vi "tm_getnextframe_a.vi"(7 "Timeout":i32=-1, 8 "error in (no error)":errorcluster, 10 "Buffer":u16[][](array[numeric]), 11 "Handle in":u32) -> (0 "error out":errorcluster, 2 "Data":u16[][](array[numeric]), 3 "Handle out":u32)   [LabVIEW 2011]
uses:
  tmcamcon.dll
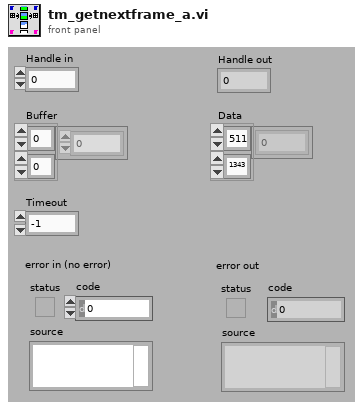
[diagram p1: front panel]
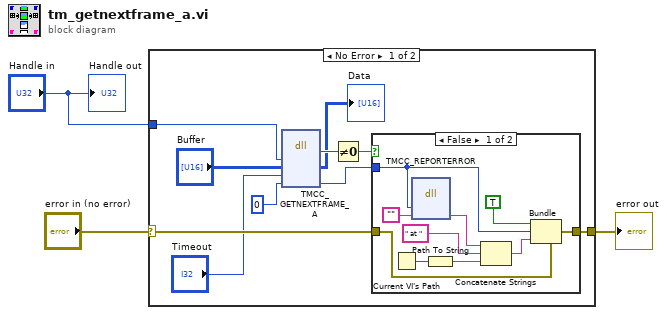
[diagram p0: block diagram]
diagram:
  n1 = case shown="No Error" "error in (no error)" {
    selector: "error in (no error)" -> [w7 w25]
    tunnel: [w6 w25] -> w2
    tunnel: "Handle in" -> [w5 _]
    frame No Error {
      n2 = dll-call lib="tmcamcon.dll" fn="TMCC_GETNEXTFRAME_A"("index"=w5, "imgarray"="Buffer", "timeout"="Timeout", "Erval"=0) -> ("return type"=w13:u32, "imgarray"=→"Data":u16[][], "Erval"=w8:i32)  [unwired: 5 in, 2 out]
      n3 = Not Equal To 0?(x=w13) -> (x != 0?=w9:bool)
      n4 = case shown="False" w9 {
        tunnel: w7 -> [w23 w24]
        tunnel: [w22 w24] -> w6
        tunnel: w8 -> [w16 _]
        frame False {
          n5 = Current VI's Path() -> (path=w21:path)
          n6 = dll-call lib="tmcamcon.dll" fn="TMCC_REPORTERROR"("error"=w16, "buf"="") -> ("buf"=w15:string)  [unwired: 5 in, 2 out]
          n7 = Path To String(path=w21) -> (string=w17:string)
          n8 = Concatenate Strings(w15, " at ", w17) -> (w20:string)
          n9 = Bundle(cluster=w23, "status"=TRUE, "code"=w16, "source"=w20) -> (w22:errorcluster)
        }
        frame True {
        }
      }
    }
    frame Error {
    }
  }
  "error out" <- w2
  "Handle out" <- "Handle in"
